vi "search.vi"(1 "Byte":u8, 2 "Buffer":string) -> (0 "Index":i32)   [LabVIEW 2022 SP3]
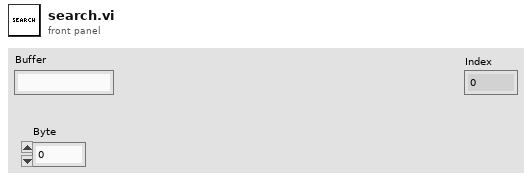
[diagram p1: front panel]
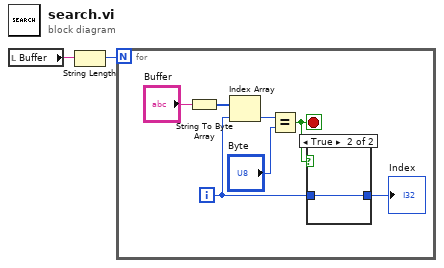
[diagram p0: block diagram]
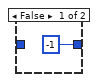
[diagram p2: hidden frame]
diagram:
  n1 = local read "Buffer"() -> (w1:string)
  n2 = String Length(string=w1) -> (length=w2:i32)
  n3 = for {
    N: w2 -> [_]
    i -> [w3]
    stop <- w5 stop-if-true
    n4 = String To Byte Array(string="Buffer") -> (unsigned byte array=w8:u8[])
    n5 = Index Array(array=w8, index=w3) -> (element=w6:u8)
    n6 = Equal?(x=w6, y="Byte") -> (x = y?=w5:bool)
    n7 = case shown="True" w5 {
      tunnel: [-1 w11] -> w4
      tunnel: w3 -> [_ w11]
      frame False {
      }
      frame True {
      }
    }
    "Index" <- w4
  }
